vi "Fetch Measurement-Sweep.vi"(8 "error in (no error)":errorcluster, 10 "Measure Call Context in":refnum<class "Measure Call Context.lvclass">, 11 "Sweep fetch measurement control":T1) -> (0 "error out":errorcluster, 3 "Sweep fetch measurement":T1)   [LabVIEW 2021, in "Sweep_Channel Ganging.lvlib"]
uses:
  Sweep_Channel Ganging.lvlib
  <vilib>/Plug-In SDKs/Measurements/Measure Call Context/Measure Call Context.lvclass
  shared subVIs/ctl/NIDCPower_channel_ganging - ctl - ganged config.ctl
  shared subVIs/ctl/NIDCPower_channel_ganging - ctl - channel mode.ctl
  shared subVIs/ctl/NIDCPower_channel_ganging - ctl - ganged session.ctl
  Measurement Results.ctl
  ctl/Sweep fetch measurement control.ctl
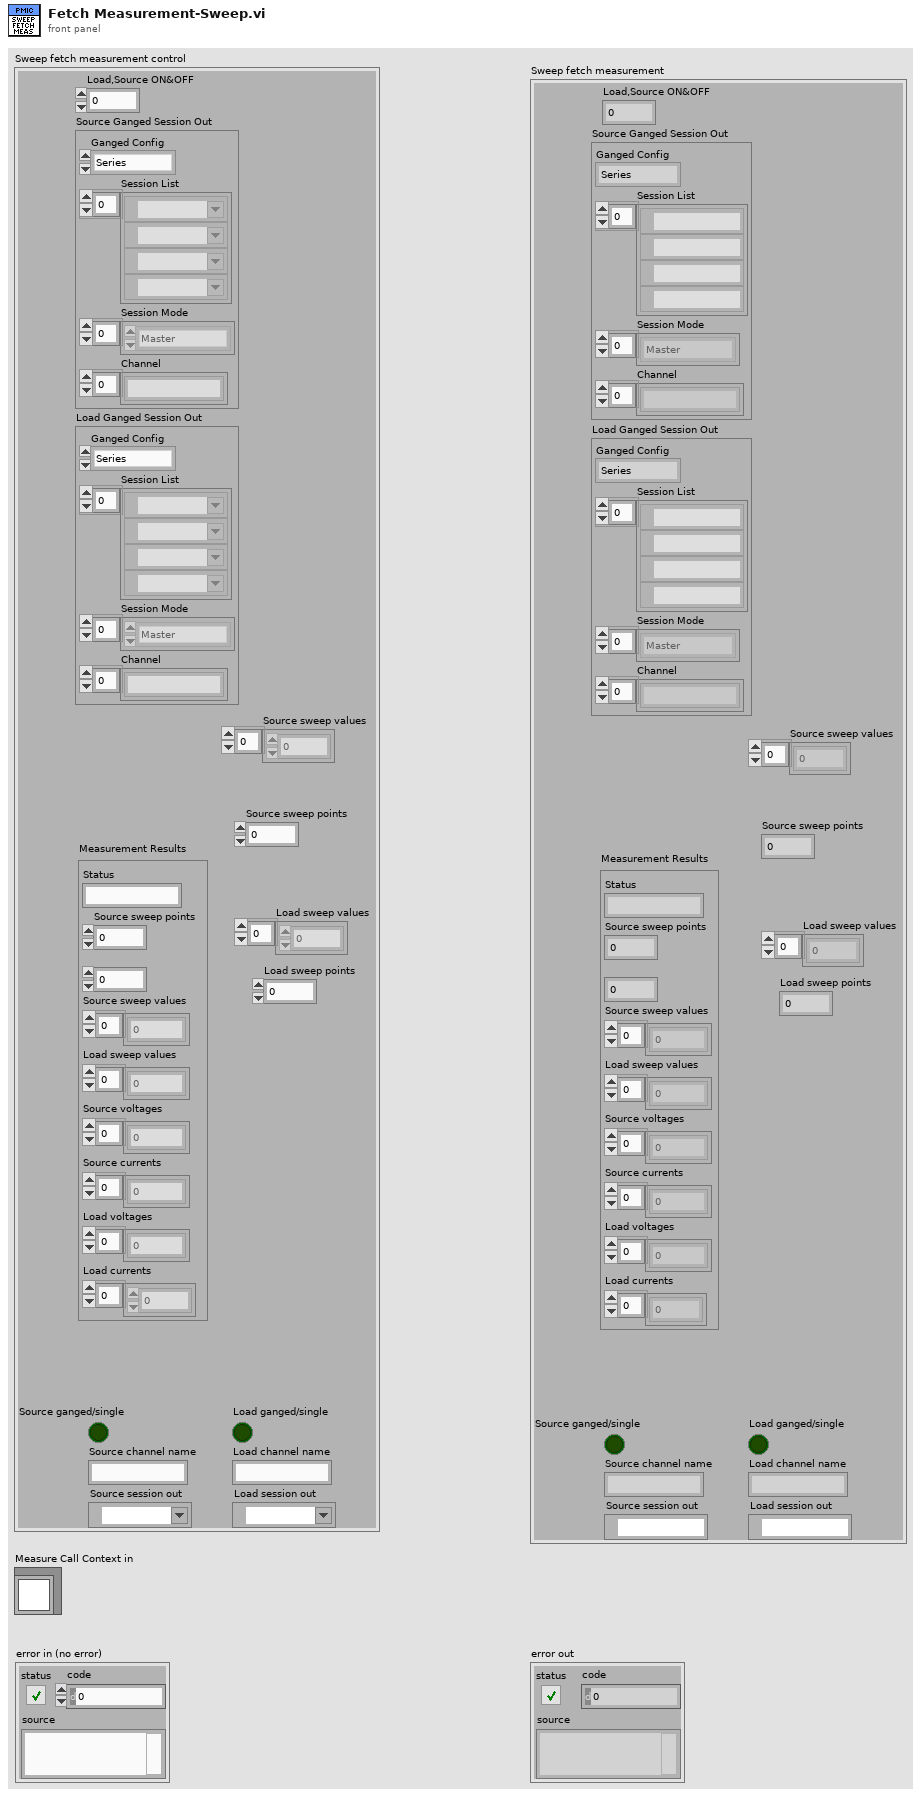
[diagram p1: front panel]
types:
  T1 = typedef "Sweep_Channel Ganging.lvlib/Sweep fetch measurement control.ctl" = cluster{"Load,Source ON&OFF":u32, "Source Ganged Session Out":T2, "Load Ganged Session Out":T2, "Source sweep values":dbl[], "Source sweep points":i32, "Load sweep values":dbl[], "Load sweep points":i32, "Measurement Results":T5, "Load ganged/single":bool, "Source ganged/single":bool, "Source channel name":string, "Load channel name":string, "Source session out":refnum<k15>, "Load session out":refnum<k15>}
  T2 = typedef "NIDCPower_channel_ganging - ctl - ganged session.ctl" = cluster{"Ganged Config":T3, "Session List":refnum<k15>[], "Session Mode":T4[], "Channel":string[]}
  T3 = typedef "NIDCPower_channel_ganging - ctl - ganged config.ctl" = enum32{"Series", "Parallel", "Manual"}
  T4 = typedef "NIDCPower_channel_ganging - ctl - channel mode.ctl" = enum32{"Master", "Slave", "Slave - Inverted"}
  T5 = typedef "Sweep_Channel Ganging.lvlib/Measurement Results.ctl" = cluster{"Status":string, "Source sweep points":i32, "Load sweep points":i32, "Source sweep values":dbl[], "Load sweep values":dbl[], "Source voltages":dbl[], "Source currents":dbl[], "Load voltages":dbl[], "Load currents":dbl[]}
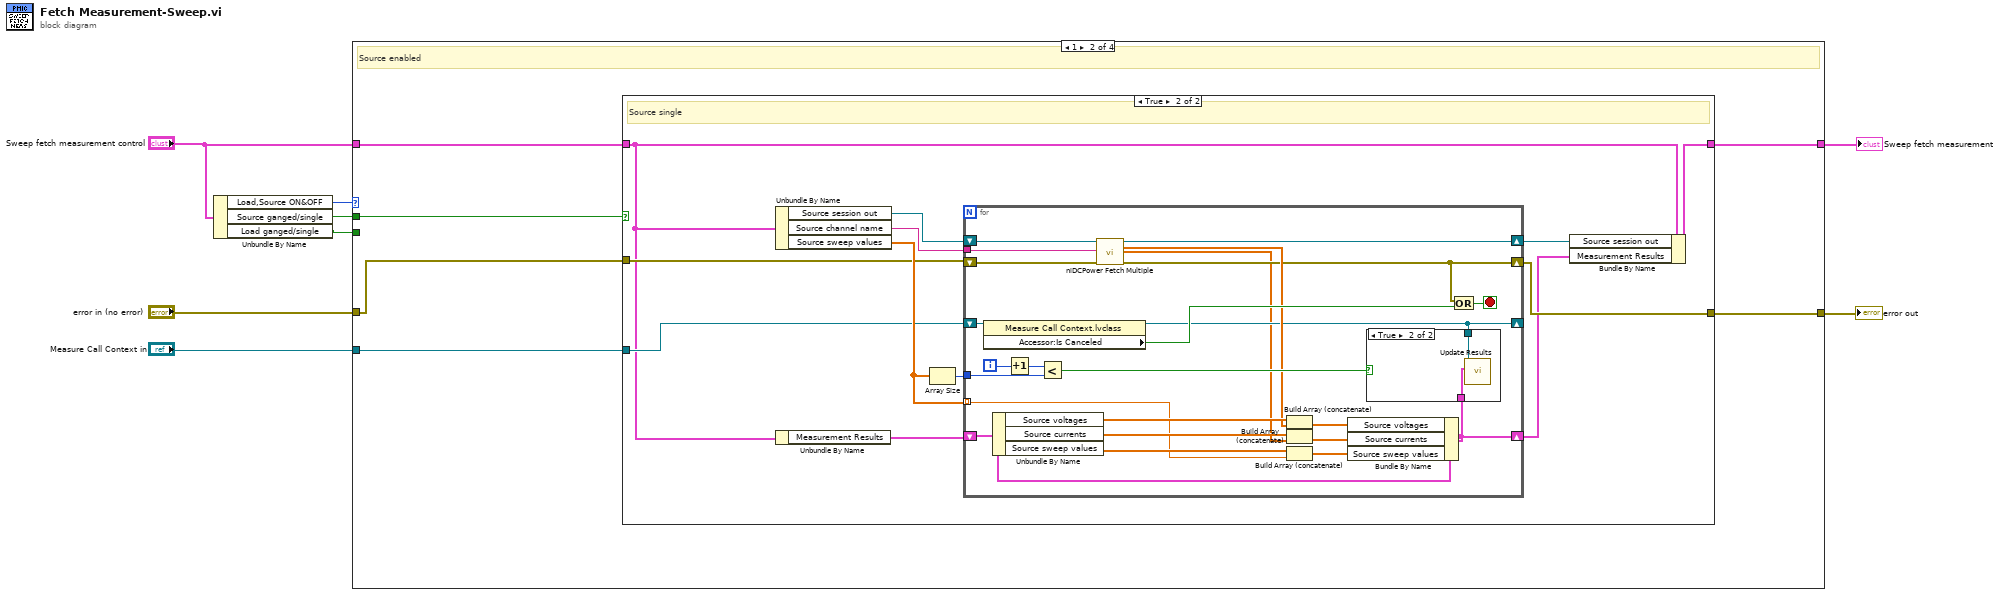
[diagram p0: block diagram]
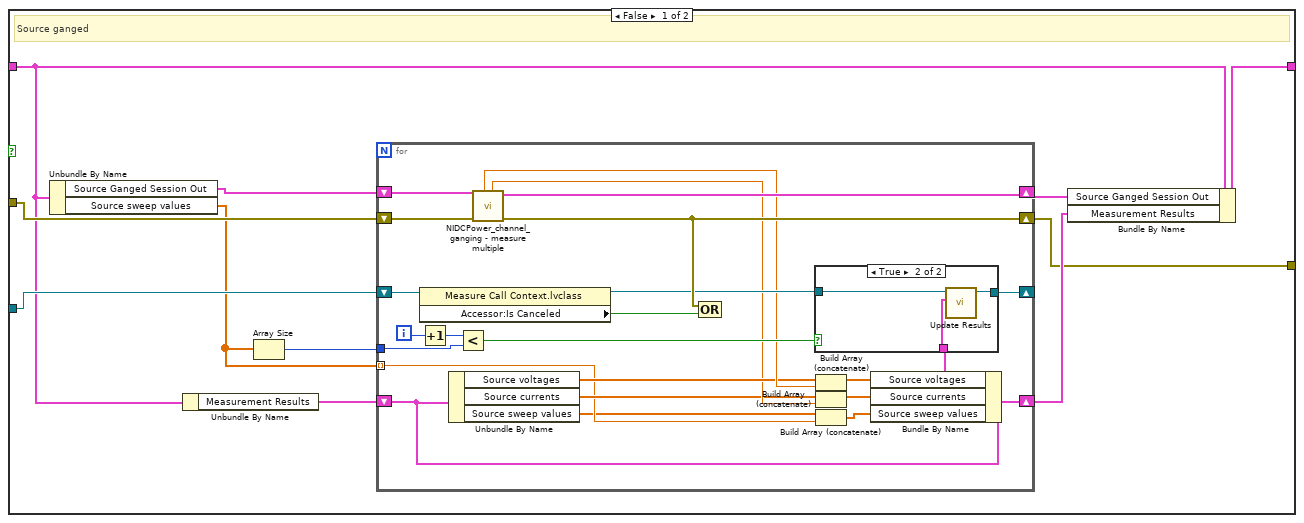
[diagram p3: hidden frame]
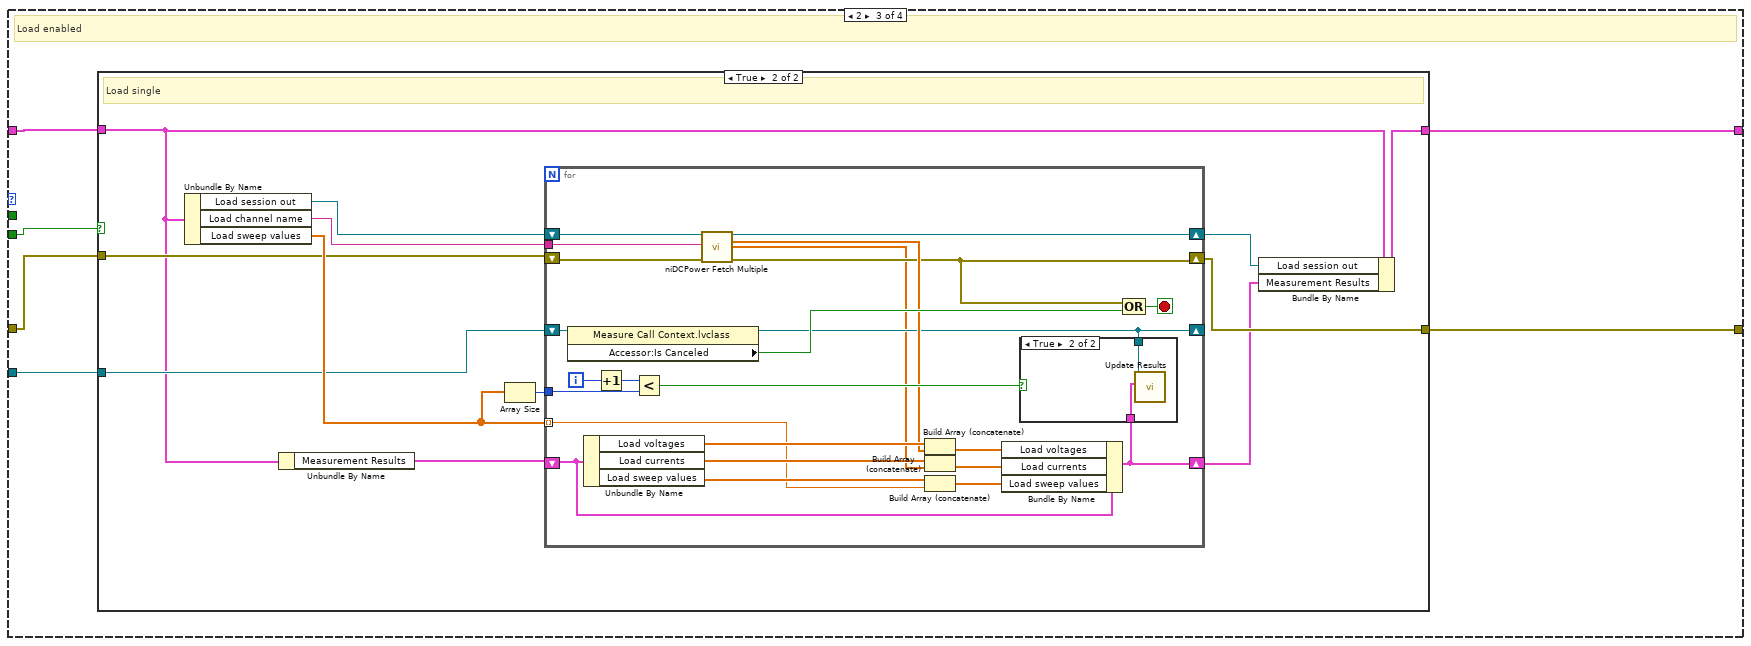
[diagram p6: hidden frame]
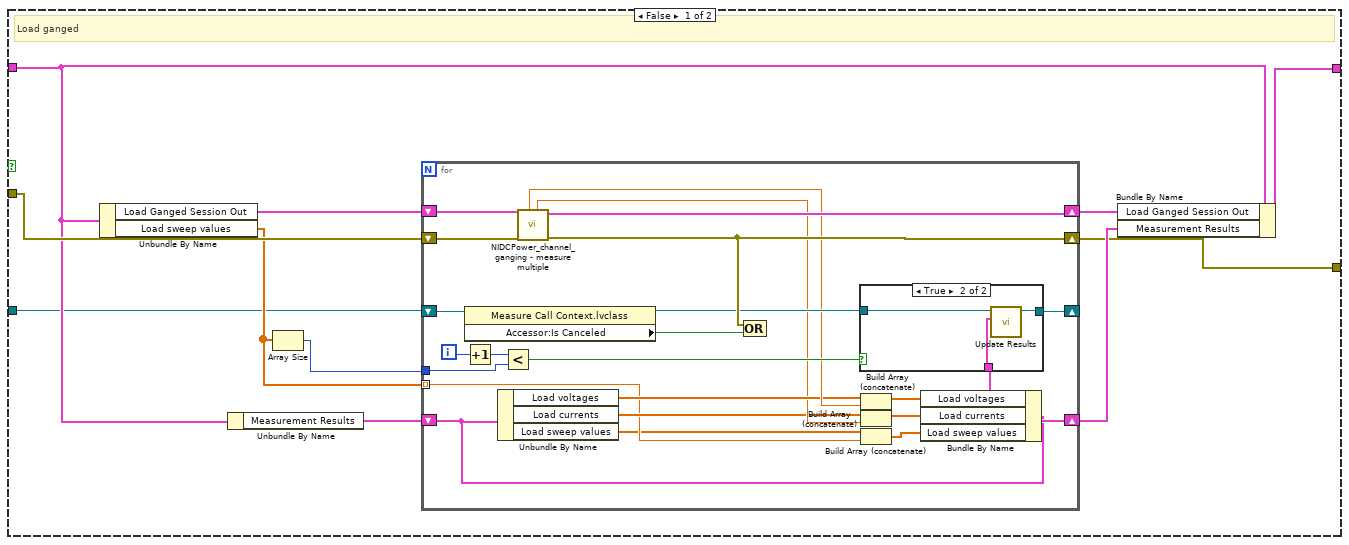
[diagram p7: hidden frame]
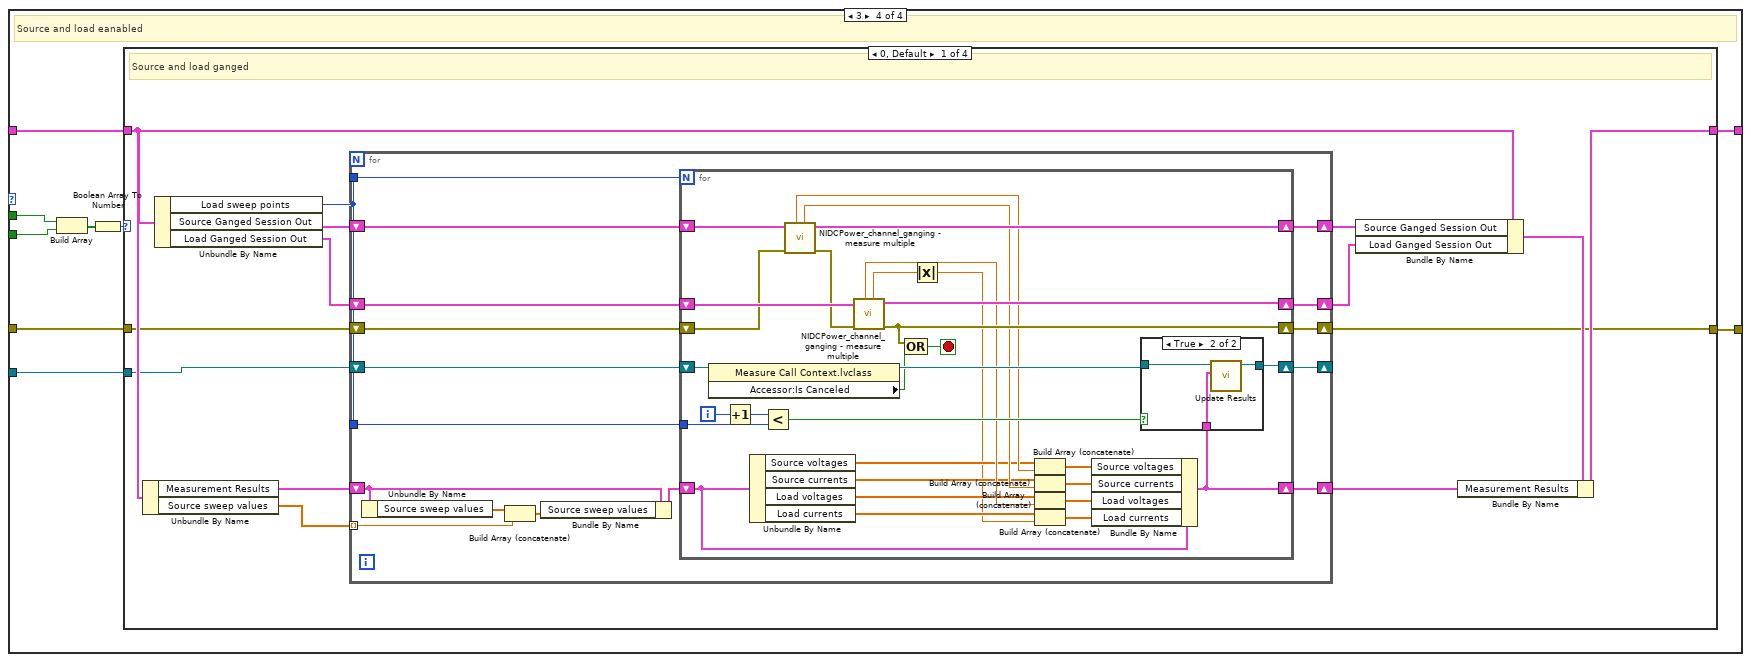
[diagram p10: hidden frame]
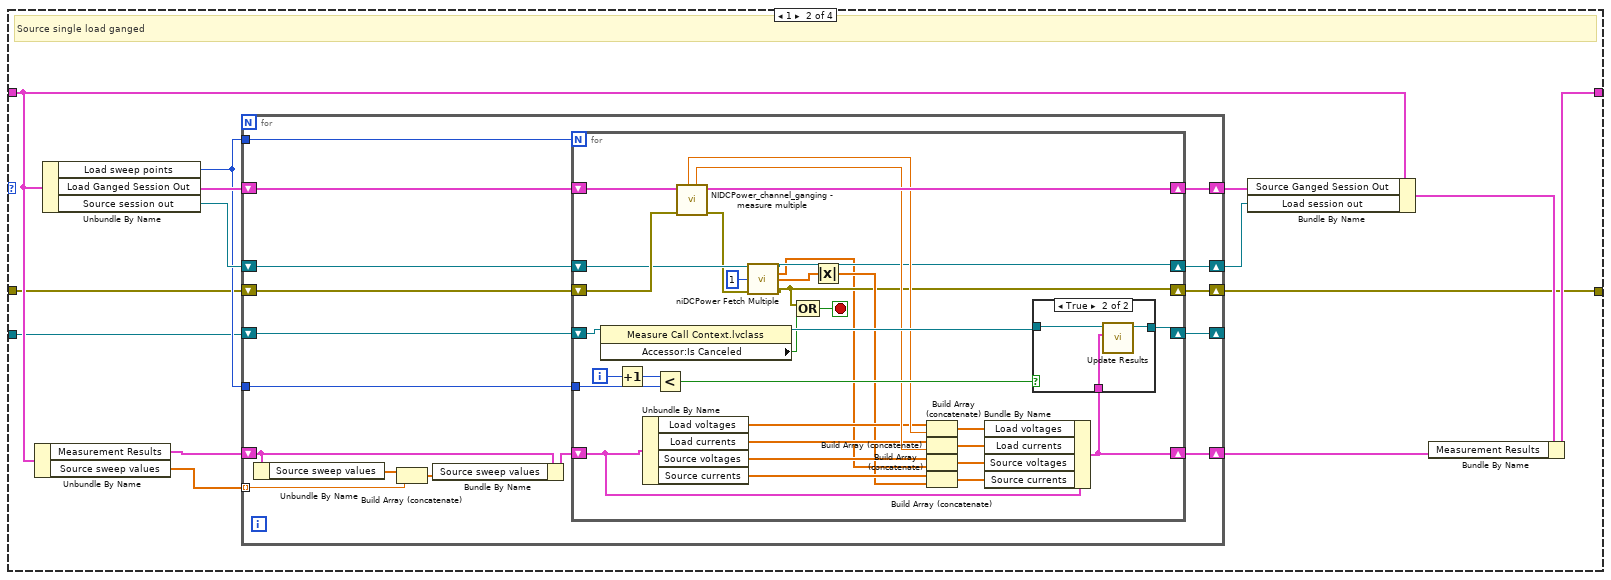
[diagram p12: hidden frame]
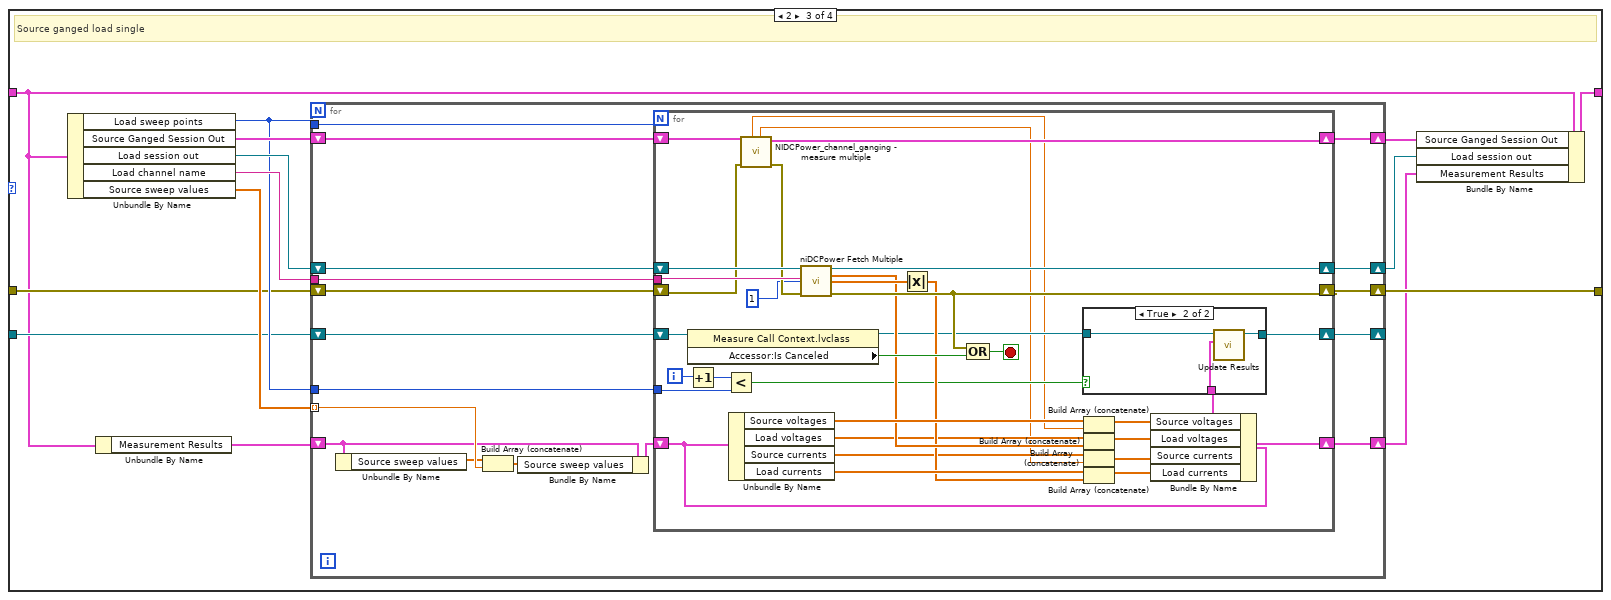
[diagram p14: hidden frame]
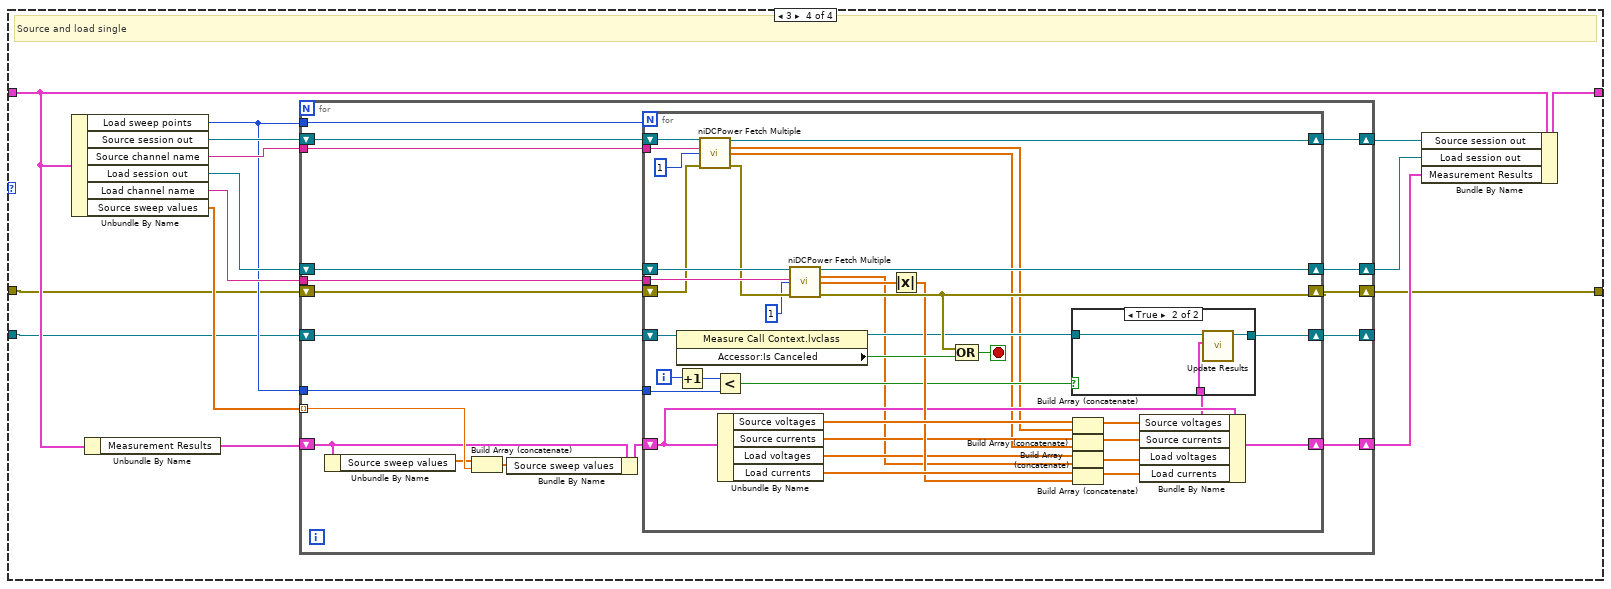
[diagram p16: hidden frame]
diagram:
  n1 = Unbundle By Name("Sweep fetch measurement control") -> ("Load,Source ON&OFF"=w4:u32, "Source ganged/single"=w3:bool, "Load ganged/single"=w2:bool)
  n2 = case shown="1" w4 {
    tunnel: "Sweep fetch measurement control" -> [w10 w15 w96 w183]
    tunnel: [w10 w12 w94 w182] -> w1
    tunnel: "Measure Call Context in" -> [_ w13 w95 w181]
    tunnel: [w9 w11 w93 w180] -> w7
    tunnel: "error in (no error)" -> [w9 w16 w98 w179]
    tunnel: w3 -> [_ w14 _ w177]
    tunnel: w2 -> [_ _ w97 w176]
    frame 0, Default {
      # "both disabled"
    }
    frame 1 {
      # "Source enabled"
      n3 = case shown="True" w14 {
        tunnel: w16 -> [w25 w62]
        tunnel: w15 -> [w21 w58]
        tunnel: w13 -> [w24 w60]
        tunnel: [w18 w57] -> w12
        tunnel: [w17 w59] -> w11
        frame False {
          # "Source ganged"
          n4 = Unbundle By Name(w21) -> ("Source Ganged Session Out"=w27:T2, "Source sweep values"=w23:dbl[])
          n5 = Unbundle By Name(w21) -> ("Measurement Results"=w20:T5)
          n6 = Array Size(array=w23) -> (size(s)=w22:i32)
          n7 = for {
            shift-right: [w49] -> w17
            shift-left: w25 -> [w50]
            shift-right: [w48] -> w26
            shift-left: w27 -> [w47]
            shift-right: [w45] -> _
            shift-left: w24 -> [w46]
            shift-right: [w44] -> w19
            shift-left: w20 -> [w34]
            tunnel: w23 -> [w30] mode=indexing
            tunnel: w22 -> [w36]
            i -> [w35]
            n8 = property class="Measure Call Context.lvclass"(reference=w46) -> (reference out=w41:refnum<class "Measure Call Context.lvclass">, "Accessor:Is Canceled"=w43:bool)  [unwired: 1 in, 1 out]
            n9 = Increment(x=w35) -> (x+1=w42:i32)
            n10 = Unbundle By Name(w34) -> ("Source voltages"=w33:dbl[], "Source currents"=w31:dbl[], "Source sweep values"=w29:dbl[])
            n11 = Less?(x=w42, y=w36) -> (x < y?=w40:bool)
            n12 = call "NIDCPower_channel_ganging - measure multiple.vi"("error in (no error)"=w50, "Ganged Session In"=w47) -> ("error out"=w49:errorcluster, "Ganged Session Out"=w48:T2, "ganged current measurement"=w32:dbl, "ganged voltage measurement"=w37:dbl)  [unwired: 2 in, 4 out]
            n13 = Compound Arithmetic op=OR(w49, w43) -> ()  [unwired: 1 out]
            n14 = Build Array (concatenate)(w33, w37) -> (w39:dbl[])
            n15 = Build Array (concatenate)(w31, w32) -> (w38:dbl[])
            n16 = Build Array (concatenate)(w29, w30) -> (w28:dbl[])
            n17 = Bundle By Name(cluster=w34, "Source voltages"=w39, "Source currents"=w38, "Source sweep values"=w28) -> (w44:T5)
            n18 = case shown="True" w40 {
              tunnel: w41 -> [w51 w54]
              tunnel: [w51 w53] -> w45
              tunnel: w44 -> [_ w52]
              frame False {
              }
              frame True {
                n19 = call <vilib>:"Update Results.vi"("measurement results"=w52, "measure call context in"=w54) -> ("measure call context out"=w53:refnum<class "Measure Call Context.lvclass">)  [unwired: 8 in, 1 out]
              }
            }
          }
          n20 = Bundle By Name(cluster=w21, "Source Ganged Session Out"=w26, "Measurement Results"=w19) -> (w18:T1)
        }
        frame True {
          # "Source single"
          n21 = Unbundle By Name(w58) -> ("Source session out"=w66:refnum<k15>, "Source channel name"=w65:string, "Source sweep values"=w64:dbl[])
          n22 = Unbundle By Name(w58) -> ("Measurement Results"=w61:T5)
          n23 = Array Size(array=w64) -> (size(s)=w63:i32)
          n24 = for {
            shift-right: [w71] -> w59
            shift-left: w62 -> [w88]
            shift-right: [w89] -> w56
            shift-left: w66 -> [w90]
            shift-right: [w80] -> w55
            shift-left: w61 -> [w81]
            shift-right: [w76] -> _
            shift-left: w60 -> [w77]
            tunnel: w65 -> [w75]
            tunnel: w64 -> [w67] mode=indexing
            tunnel: w63 -> [w74]
            i -> [w87]
            stop <- w83 stop-if-true
            n25 = property class="Measure Call Context.lvclass"(reference=w77) -> (reference out=w76:refnum<class "Measure Call Context.lvclass">, "Accessor:Is Canceled"=w84:bool)  [unwired: 1 in, 1 out]
            n26 = Unbundle By Name(w81) -> ("Source voltages"=w82:dbl[], "Source currents"=w73:dbl[], "Source sweep values"=w72:dbl[])
            n27 = Increment(x=w87) -> (x+1=w86:i32)
            n28 = Less?(x=w86, y=w74) -> (x < y?=w85:bool)
            n29 = call <instrlib>:"niDCPower Fetch Multiple.vi"("instrument handle"=w90, "channel name"=w75, "error in (no error)"=w88) -> ("instrument handle out"=w89:refnum<k15>, "voltage measurements"=w79:dbl[], "current measurements"=w68:dbl[], "error out"=w71:errorcluster)  [unwired: 2 in, 7 out]
            n30 = Build Array (concatenate)(w82, w79) -> (w69:dbl[])
            n31 = Build Array (concatenate)(w73, w68) -> (w70:dbl[])
            n32 = Build Array (concatenate)(w72, w67) -> (w78:dbl[])
            n33 = Bundle By Name(cluster=w81, "Source voltages"=w69, "Source currents"=w70, "Source sweep values"=w78) -> (w80:T5)
            n34 = case shown="True" w85 {
              tunnel: w76 -> [_ w92]
              tunnel: w80 -> [_ w91]
              frame False {
              }
              frame True {
                n35 = call <vilib>:"Update Results.vi"("measurement results"=w91, "measure call context in"=w92) -> ()  [unwired: 8 in, 2 out]
              }
            }
            n36 = Compound Arithmetic op=OR(w71, w84) -> (w83:bool)
          }
          n37 = Bundle By Name(cluster=w58, "Source session out"=w56, "Measurement Results"=w55) -> (w57:T1)
        }
      }
    }
    frame 2 {
      # "Load enabled"
      n38 = case shown="True" w97 {
        tunnel: w98 -> [w107 w144]
        tunnel: w96 -> [w104 w140]
        tunnel: w95 -> [w99 w142]
        tunnel: [w101 w139] -> w94
        tunnel: [w100 w141] -> w93
        frame False {
          # "Load ganged"
          n39 = Unbundle By Name(w104) -> ("Load Ganged Session Out"=w109:T2, "Load sweep values"=w106:dbl[])
          n40 = Unbundle By Name(w104) -> ("Measurement Results"=w103:T5)
          n41 = Array Size(array=w106) -> (size(s)=w105:i32)
          n42 = for {
            shift-right: [w131] -> w100
            shift-left: w107 -> [w132]
            shift-right: [w130] -> w108
            shift-left: w109 -> [w129]
            shift-right: [w127] -> _
            shift-left: w99 -> [w128]
            shift-right: [w126] -> w102
            shift-left: w103 -> [w116]
            tunnel: w106 -> [w112] mode=indexing
            tunnel: w105 -> [w118]
            i -> [w117]
            n43 = property class="Measure Call Context.lvclass"(reference=w128) -> (reference out=w123:refnum<class "Measure Call Context.lvclass">, "Accessor:Is Canceled"=w125:bool)  [unwired: 1 in, 1 out]
            n44 = Increment(x=w117) -> (x+1=w124:i32)
            n45 = Unbundle By Name(w116) -> ("Load voltages"=w115:dbl[], "Load currents"=w113:dbl[], "Load sweep values"=w111:dbl[])
            n46 = Less?(x=w124, y=w118) -> (x < y?=w122:bool)
            n47 = call "NIDCPower_channel_ganging - measure multiple.vi"("error in (no error)"=w132, "Ganged Session In"=w129) -> ("error out"=w131:errorcluster, "Ganged Session Out"=w130:T2, "ganged current measurement"=w114:dbl, "ganged voltage measurement"=w119:dbl)  [unwired: 2 in, 4 out]
            n48 = Compound Arithmetic op=OR(w131, w125) -> ()  [unwired: 1 out]
            n49 = Build Array (concatenate)(w115, w119) -> (w121:dbl[])
            n50 = Build Array (concatenate)(w113, w114) -> (w120:dbl[])
            n51 = Build Array (concatenate)(w111, w112) -> (w110:dbl[])
            n52 = Bundle By Name(cluster=w116, "Load voltages"=w121, "Load currents"=w120, "Load sweep values"=w110) -> (w126:T5)
            n53 = case shown="True" w122 {
              tunnel: w123 -> [w133 w136]
              tunnel: [w133 w135] -> w127
              tunnel: w126 -> [_ w134]
              frame False {
              }
              frame True {
                n54 = call <vilib>:"Update Results.vi"("measurement results"=w134, "measure call context in"=w136) -> ("measure call context out"=w135:refnum<class "Measure Call Context.lvclass">)  [unwired: 8 in, 1 out]
              }
            }
          }
          n55 = Bundle By Name(cluster=w104, "Load Ganged Session Out"=w108, "Measurement Results"=w102) -> (w101:T1)
        }
        frame True {
          # "Load single"
          n56 = Unbundle By Name(w140) -> ("Load session out"=w148:refnum<k15>, "Load channel name"=w147:string, "Load sweep values"=w146:dbl[])
          n57 = Unbundle By Name(w140) -> ("Measurement Results"=w143:T5)
          n58 = Array Size(array=w146) -> (size(s)=w145:i32)
          n59 = for {
            shift-right: [w153] -> w141
            shift-left: w144 -> [w170]
            shift-right: [w171] -> w138
            shift-left: w148 -> [w172]
            shift-right: [w162] -> w137
            shift-left: w143 -> [w163]
            shift-right: [w158] -> _
            shift-left: w142 -> [w159]
            tunnel: w147 -> [w157]
            tunnel: w146 -> [w149] mode=indexing
            tunnel: w145 -> [w156]
            i -> [w169]
            stop <- w165 stop-if-true
            n60 = property class="Measure Call Context.lvclass"(reference=w159) -> (reference out=w158:refnum<class "Measure Call Context.lvclass">, "Accessor:Is Canceled"=w166:bool)  [unwired: 1 in, 1 out]
            n61 = Unbundle By Name(w163) -> ("Load voltages"=w164:dbl[], "Load currents"=w155:dbl[], "Load sweep values"=w154:dbl[])
            n62 = Increment(x=w169) -> (x+1=w168:i32)
            n63 = Less?(x=w168, y=w156) -> (x < y?=w167:bool)
            n64 = call <instrlib>:"niDCPower Fetch Multiple.vi"("instrument handle"=w172, "channel name"=w157, "error in (no error)"=w170) -> ("instrument handle out"=w171:refnum<k15>, "voltage measurements"=w161:dbl[], "current measurements"=w150:dbl[], "error out"=w153:errorcluster)  [unwired: 2 in, 7 out]
            n65 = Build Array (concatenate)(w164, w161) -> (w151:dbl[])
            n66 = Build Array (concatenate)(w155, w150) -> (w152:dbl[])
            n67 = Build Array (concatenate)(w154, w149) -> (w160:dbl[])
            n68 = Bundle By Name(cluster=w163, "Load voltages"=w151, "Load currents"=w152, "Load sweep values"=w160) -> (w162:T5)
            n69 = case shown="True" w167 {
              tunnel: w158 -> [_ w174]
              tunnel: w162 -> [_ w173]
              frame False {
              }
              frame True {
                n70 = call <vilib>:"Update Results.vi"("measurement results"=w173, "measure call context in"=w174) -> ()  [unwired: 8 in, 2 out]
              }
            }
            n71 = Compound Arithmetic op=OR(w153, w166) -> (w165:bool)
          }
          n72 = Bundle By Name(cluster=w140, "Load session out"=w138, "Measurement Results"=w137) -> (w139:T1)
        }
      }
    }
    frame 3 {
      # "Source and load eanabled"
      n73 = Build Array(w177, w176) -> (w178:bool[])
      n74 = Boolean Array To Number(Boolean array=w178) -> (number=w175:u32)
      n75 = case shown="0, Default" w175 {
        tunnel: w183 -> [w193 w253 w319 w387]
        tunnel: [w189 w254 w318 w383] -> w182
        tunnel: w181 -> [w186 w252 w322 w385]
        tunnel: [w185 w250 w320 w384] -> w180
        tunnel: w179 -> [w184 w251 w323 w386]
        frame 0, Default {
          # "Source and load ganged"
          n76 = Unbundle By Name(w193) -> ("Measurement Results"=w187:T5, "Source sweep values"=w197:dbl[])
          n77 = Unbundle By Name(w193) -> ("Load sweep points"=w190:i32, "Source Ganged Session Out"=w191:T2, "Load Ganged Session Out"=w192:T2)
          n78 = for {
            shift-right: [w212] -> w185
            shift-left: w184 -> [w213]
            shift-right: [w210] -> w195
            shift-left: w192 -> [w211]
            shift-right: [w208] -> w194
            shift-left: w191 -> [w209]
            shift-right: [w206] -> _
            shift-left: w186 -> [w207]
            shift-right: [w205] -> w188
            shift-left: w187 -> [w200]
            tunnel: w190 -> [w204]
            tunnel: w190 -> [w203]
            tunnel: w197 -> [w198] mode=indexing
            n79 = Unbundle By Name(w200) -> ("Source sweep values"=w202:dbl[])
            n80 = Build Array (concatenate)(w202, w198) -> (w201:dbl[])
            n81 = Bundle By Name(cluster=w200, "Source sweep values"=w201) -> (w199:T5)
            n82 = for {
              N: w203 -> [_]
              shift-right: [w233] -> w212
              shift-left: w213 -> [w242]
              shift-right: [w243] -> w210
              shift-left: w211 -> [w244]
              shift-right: [w239] -> w208
              shift-left: w209 -> [w240]
              shift-right: [w236] -> w206
              shift-left: w207 -> [w238]
              shift-right: [w229] -> w205
              shift-left: w199 -> [w232]
              tunnel: w204 -> [w219]
              i -> [w227]
              stop <- w235 stop-if-true
              n83 = property class="Measure Call Context.lvclass"(reference=w238) -> (reference out=w237:refnum<class "Measure Call Context.lvclass">, "Accessor:Is Canceled"=w234:bool)  [unwired: 1 in, 1 out]
              n84 = Increment(x=w227) -> (x+1=w228:i32)
              n85 = Unbundle By Name(w232) -> ("Source voltages"=w218:dbl[], "Source currents"=w217:dbl[], "Load voltages"=w216:dbl[], "Load currents"=w215:dbl[])
              n86 = Less?(x=w228, y=w219) -> (x < y?=w226:bool)
              n87 = call "NIDCPower_channel_ganging - measure multiple.vi"("error in (no error)"=w242, "Ganged Session In"=w240) -> ("error out"=w241:errorcluster, "Ganged Session Out"=w239:T2, "ganged current measurement"=w224:dbl, "ganged voltage measurement"=w225:dbl)  [unwired: 2 in, 4 out]
              n88 = call "NIDCPower_channel_ganging - measure multiple.vi"("error in (no error)"=w241, "Ganged Session In"=w244) -> ("error out"=w233:errorcluster, "Ganged Session Out"=w243:T2, "ganged current measurement"=w222:dbl, "ganged voltage measurement"=w223:dbl)  [unwired: 2 in, 4 out]
              n89 = Compound Arithmetic op=OR(w233, w234) -> (w235:bool)
              n90 = Absolute Value(x=w222) -> (abs(x)=w214:dbl)
              n91 = Build Array (concatenate)(w218, w225) -> (w231:dbl[])
              n92 = Build Array (concatenate)(w217, w224) -> (w230:dbl[])
              n93 = Build Array (concatenate)(w216, w223) -> (w221:dbl[])
              n94 = Build Array (concatenate)(w215, w214) -> (w220:dbl[])
              n95 = Bundle By Name(cluster=w232, "Source voltages"=w231, "Source currents"=w230, "Load voltages"=w221, "Load currents"=w220) -> (w229:T5)
              n96 = case shown="True" w226 {
                tunnel: w229 -> [_ w248]
                tunnel: w237 -> [w245 w247]
                tunnel: [w245 w246] -> w236
                frame False {
                }
                frame True {
                  n97 = call <vilib>:"Update Results.vi"("measurement results"=w248, "measure call context in"=w247) -> ("measure call context out"=w246:refnum<class "Measure Call Context.lvclass">)  [unwired: 8 in, 1 out]
                }
              }
            }
          }
          n98 = Bundle By Name(cluster=w193, "Source Ganged Session Out"=w194, "Load Ganged Session Out"=w195) -> (w196:T1)
          n99 = Bundle By Name(cluster=w196, "Measurement Results"=w188) -> (w189:T1)
        }
        frame 1 {
          # "Source single load ganged"
          n100 = Unbundle By Name(w253) -> ("Measurement Results"=w255:T5, "Source sweep values"=w262:dbl[])
          n101 = Unbundle By Name(w253) -> ("Load sweep points"=w257:i32, "Load Ganged Session Out"=w258:T2, "Source session out"=w259:refnum<k15>)
          n102 = for {
            shift-right: [w277] -> w250
            shift-left: w251 -> [w278]
            shift-right: [w275] -> w249
            shift-left: w259 -> [w276]
            shift-right: [w273] -> w260
            shift-left: w258 -> [w274]
            shift-right: [w271] -> _
            shift-left: w252 -> [w272]
            shift-right: [w270] -> w256
            shift-left: w255 -> [w265]
            tunnel: w257 -> [w269]
            tunnel: w257 -> [w268]
            tunnel: w262 -> [w263] mode=indexing
            n103 = Unbundle By Name(w265) -> ("Source sweep values"=w267:dbl[])
            n104 = Build Array (concatenate)(w267, w263) -> (w266:dbl[])
            n105 = Bundle By Name(cluster=w265, "Source sweep values"=w266) -> (w264:T5)
            n106 = for {
              N: w268 -> [_]
              shift-right: [w282] -> w277
              shift-left: w278 -> [w310]
              shift-right: [w284] -> w275
              shift-left: w276 -> [w285]
              shift-right: [w308] -> w273
              shift-left: w274 -> [w309]
              shift-right: [w305] -> w271
              shift-left: w272 -> [w307]
              shift-right: [w299] -> w270
              shift-left: w264 -> [w302]
              tunnel: w269 -> [w291]
              i -> [w297]
              stop <- w304 stop-if-true
              n107 = property class="Measure Call Context.lvclass"(reference=w307) -> (reference out=w306:refnum<class "Measure Call Context.lvclass">, "Accessor:Is Canceled"=w303:bool)  [unwired: 1 in, 1 out]
              n108 = Increment(x=w297) -> (x+1=w298:i32)
              n109 = Unbundle By Name(w302) -> ("Load voltages"=w290:dbl[], "Load currents"=w289:dbl[], "Source voltages"=w288:dbl[], "Source currents"=w287:dbl[])
              n110 = Less?(x=w298, y=w291) -> (x < y?=w296:bool)
              n111 = call "NIDCPower_channel_ganging - measure multiple.vi"("error in (no error)"=w310, "Ganged Session In"=w309) -> ("error out"=w283:errorcluster, "Ganged Session Out"=w308:T2, "ganged current measurement"=w294:dbl, "ganged voltage measurement"=w295:dbl)  [unwired: 2 in, 4 out]
              n112 = call <instrlib>:"niDCPower Fetch Multiple.vi"("instrument handle"=w285, "count (1)"=1, "error in (no error)"=w283) -> ("instrument handle out"=w284:refnum<k15>, "voltage measurements"=w281:dbl[], "current measurements"=w280:dbl[], "error out"=w282:errorcluster)  [unwired: 2 in, 7 out]
              n113 = Compound Arithmetic op=OR(w282, w303) -> (w304:bool)
              n114 = Absolute Value(x=w280) -> (abs(x)=w286:dbl[])
              n115 = Build Array (concatenate)(w290, w295) -> (w301:dbl[])
              n116 = Build Array (concatenate)(w289, w294) -> (w300:dbl[])
              n117 = Build Array (concatenate)(w288, w281) -> (w293:dbl[])
              n118 = Build Array (concatenate)(w287, w286) -> (w292:dbl[])
              n119 = Bundle By Name(cluster=w302, "Load voltages"=w301, "Load currents"=w300, "Source voltages"=w293, "Source currents"=w292) -> (w299:T5)
              n120 = case shown="True" w296 {
                tunnel: w299 -> [_ w314]
                tunnel: w306 -> [w311 w313]
                tunnel: [w311 w312] -> w305
                frame False {
                }
                frame True {
                  n121 = call <vilib>:"Update Results.vi"("measurement results"=w314, "measure call context in"=w313) -> ("measure call context out"=w312:refnum<class "Measure Call Context.lvclass">)  [unwired: 8 in, 1 out]
                }
              }
            }
          }
          n122 = Bundle By Name(cluster=w253, "Source Ganged Session Out"=w260, "Load session out"=w249) -> (w261:T1)
          n123 = Bundle By Name(cluster=w261, "Measurement Results"=w256) -> (w254:T1)
        }
        frame 2 {
          # "Source ganged load single"
          n124 = Unbundle By Name(w319) -> ("Load sweep points"=w324:i32, "Source Ganged Session Out"=w328:T2, "Load session out"=w327:refnum<k15>, "Load channel name"=w326:string, "Source sweep values"=w325:dbl[])
          n125 = Unbundle By Name(w319) -> ("Measurement Results"=w321:T5)
          n126 = for {
            tunnel: w326 -> [w339]
            tunnel: w324 -> [w338]
            shift-right: [w344] -> w320
            shift-left: w323 -> [w345]
            shift-right: [w342] -> w316
            shift-left: w328 -> [w341]
            shift-right: [w343] -> w317
            shift-left: w327 -> [w340]
            shift-right: [w336] -> _
            shift-left: w322 -> [w337]
            shift-right: [w329] -> w315
            shift-left: w321 -> [w333]
            tunnel: w325 -> [w334] mode=indexing
            tunnel: w324 -> [w335]
            n127 = Unbundle By Name(w333) -> ("Source sweep values"=w330:dbl[])
            n128 = Build Array (concatenate)(w330, w334) -> (w331:dbl[])
            n129 = Bundle By Name(cluster=w333, "Source sweep values"=w331) -> (w332:T5)
            n130 = for {
              N: w338 -> [_]
              tunnel: w339 -> [w377]
              shift-right: [w378] -> w343
              shift-left: w340 -> [w376]
              shift-right: [w373] -> w344
              shift-left: w345 -> [w352]
              shift-right: [w349] -> w342
              shift-left: w341 -> [w350]
              shift-right: [w362] -> w336
              shift-left: w337 -> [w370]
              shift-right: [w353] -> w329
              shift-left: w332 -> [w354]
              tunnel: w335 -> [w361]
              i -> [w371]
              stop <- w364 stop-if-true
              n131 = property class="Measure Call Context.lvclass"(reference=w370) -> (reference out=w363:refnum<class "Measure Call Context.lvclass">, "Accessor:Is Canceled"=w374:bool)  [unwired: 1 in, 1 out]
              n132 = Increment(x=w371) -> (x+1=w372:i32)
              n133 = Less?(x=w372, y=w361) -> (x < y?=w358:bool)
              n134 = Unbundle By Name(w354) -> ("Source voltages"=w367:dbl[], "Load voltages"=w359:dbl[], "Source currents"=w360:dbl[], "Load currents"=w368:dbl[])
              n135 = call "NIDCPower_channel_ganging - measure multiple.vi"("error in (no error)"=w352, "Ganged Session In"=w350) -> ("error out"=w351:errorcluster, "Ganged Session Out"=w349:T2, "ganged current measurement"=w347:dbl, "ganged voltage measurement"=w348:dbl)  [unwired: 2 in, 4 out]
              n136 = call <instrlib>:"niDCPower Fetch Multiple.vi"("instrument handle"=w376, "channel name"=w377, "count (1)"=1, "error in (no error)"=w351) -> ("instrument handle out"=w378:refnum<k15>, "voltage measurements"=w366:dbl[], "current measurements"=w375:dbl[], "error out"=w373:errorcluster)  [unwired: 1 in, 7 out]
              n137 = Absolute Value(x=w375) -> (abs(x)=w365:dbl[])
              n138 = Compound Arithmetic op=OR(w373, w374) -> (w364:bool)
              n139 = Build Array (concatenate)(w367, w348) -> (w357:dbl[])
              n140 = Build Array (concatenate)(w359, w366) -> (w356:dbl[])
              n141 = Build Array (concatenate)(w360, w347) -> (w369:dbl[])
              n142 = Build Array (concatenate)(w368, w365) -> (w355:dbl[])
              n143 = Bundle By Name(cluster=w354, "Source voltages"=w357, "Load voltages"=w356, "Source currents"=w369, "Load currents"=w355) -> (w353:T5)
              n144 = case shown="True" w358 {
                tunnel: w363 -> [w379 w382]
                tunnel: [w379 w381] -> w362
                tunnel: w353 -> [_ w380]
                frame False {
                }
                frame True {
                  n145 = call <vilib>:"Update Results.vi"("measurement results"=w380, "measure call context in"=w382) -> ("measure call context out"=w381:refnum<class "Measure Call Context.lvclass">)  [unwired: 8 in, 1 out]
                }
              }
            }
          }
          n146 = Bundle By Name(cluster=w319, "Source Ganged Session Out"=w316, "Load session out"=w317, "Measurement Results"=w315) -> (w318:T1)
        }
        frame 3 {
          # "Source and load single"
          n147 = Unbundle By Name(w387) -> ("Load sweep points"=w392:i32, "Source session out"=w397:refnum<k15>, "Source channel name"=w396:string, "Load session out"=w395:refnum<k15>, "Load channel name"=w394:string, "Source sweep values"=w393:dbl[])
          n148 = Unbundle By Name(w387) -> ("Measurement Results"=w391:T5)
          n149 = for {
            tunnel: w396 -> [w410]
            tunnel: w394 -> [w408]
            tunnel: w392 -> [w407]
            shift-right: [w414] -> w384
            shift-left: w386 -> [w415]
            shift-right: [w412] -> w389
            shift-left: w397 -> [w411]
            shift-right: [w413] -> w390
            shift-left: w395 -> [w409]
            shift-right: [w405] -> _
            shift-left: w385 -> [w406]
            shift-right: [w398] -> w388
            shift-left: w391 -> [w402]
            tunnel: w393 -> [w403] mode=indexing
            tunnel: w392 -> [w404]
            n150 = Unbundle By Name(w402) -> ("Source sweep values"=w399:dbl[])
            n151 = Build Array (concatenate)(w399, w403) -> (w400:dbl[])
            n152 = Bundle By Name(cluster=w402, "Source sweep values"=w400) -> (w401:T5)
            n153 = for {
              N: w407 -> [_]
              tunnel: w408 -> [w449]
              tunnel: w410 -> [w422]
              shift-right: [w450] -> w413
              shift-left: w409 -> [w448]
              shift-right: [w445] -> w414
              shift-left: w415 -> [w425]
              shift-right: [w420] -> w412
              shift-left: w411 -> [w423]
              shift-right: [w435] -> w405
              shift-left: w406 -> [w442]
              shift-right: [w426] -> w398
              shift-left: w401 -> [w427]
              tunnel: w404 -> [w434]
              i -> [w443]
              stop <- w437 stop-if-true
              n154 = property class="Measure Call Context.lvclass"(reference=w442) -> (reference out=w436:refnum<class "Measure Call Context.lvclass">, "Accessor:Is Canceled"=w446:bool)  [unwired: 1 in, 1 out]
              n155 = Increment(x=w443) -> (x+1=w444:i32)
              n156 = call <instrlib>:"niDCPower Fetch Multiple.vi"("instrument handle"=w423, "channel name"=w422, "count (1)"=1, "error in (no error)"=w425) -> ("instrument handle out"=w420:refnum<k15>, "voltage measurements"=w421:dbl[], "current measurements"=w417:dbl[], "error out"=w424:errorcluster)  [unwired: 1 in, 7 out]
              n157 = Less?(x=w444, y=w434) -> (x < y?=w431:bool)
              n158 = Unbundle By Name(w427) -> ("Source voltages"=w439:dbl[], "Source currents"=w432:dbl[], "Load voltages"=w433:dbl[], "Load currents"=w440:dbl[])
              n159 = call <instrlib>:"niDCPower Fetch Multiple.vi"("instrument handle"=w448, "channel name"=w449, "count (1)"=1, "error in (no error)"=w424) -> ("instrument handle out"=w450:refnum<k15>, "voltage measurements"=w416:dbl[], "current measurements"=w447:dbl[], "error out"=w445:errorcluster)  [unwired: 1 in, 7 out]
              n160 = Absolute Value(x=w447) -> (abs(x)=w438:dbl[])
              n161 = Compound Arithmetic op=OR(w445, w446) -> (w437:bool)
              n162 = Build Array (concatenate)(w439, w421) -> (w430:dbl[])
              n163 = Build Array (concatenate)(w432, w417) -> (w429:dbl[])
              n164 = Build Array (concatenate)(w433, w416) -> (w441:dbl[])
              n165 = Build Array (concatenate)(w440, w438) -> (w428:dbl[])
              n166 = Bundle By Name(cluster=w427, "Source voltages"=w430, "Source currents"=w429, "Load voltages"=w441, "Load currents"=w428) -> (w426:T5)
              n167 = case shown="True" w431 {
                tunnel: w436 -> [w451 w454]
                tunnel: [w451 w453] -> w435
                tunnel: w426 -> [_ w452]
                frame False {
                }
                frame True {
                  n168 = call <vilib>:"Update Results.vi"("measurement results"=w452, "measure call context in"=w454) -> ("measure call context out"=w453:refnum<class "Measure Call Context.lvclass">)  [unwired: 8 in, 1 out]
                }
              }
            }
          }
          n169 = Bundle By Name(cluster=w387, "Source session out"=w389, "Load session out"=w390, "Measurement Results"=w388) -> (w383:T1)
        }
      }
    }
  }
  "error out" <- w7
  "Sweep fetch measurement" <- w1
